vi "SerialTest.vi"(8 "error in (no error)":errorcluster, 11 "ControlBoard VISA":refnum<visa-resource-name>="ControlBoard") -> (0 "error out":errorcluster, 2 "Result":string="m\r\n\r\n\r\n----------------------------------------------\r\nEPC CONTROL BOARD TEST MENU: \r\n----------------------------------------------\r\na - Report ADC Results in Counts\r\nb - Repeat Single ADC Result\r\nc - Report ADC Results in Volts\r\nd - Clear Fault bits\r\ne - Report the Fault bits\r\nf - Run EEPROM Test\r\ng - Run SRAM Test\r\nh - Run Expansion Tests\r\ni - Turn Debug LEDs on/off\r\nj - Get Digital Input Pin State\r\nk - Set Digital Output Pin State\r\nl - Set Relay Driver State\r\nn - Boot Enable Pin State\r\no - Run CAN Test\r\np - Read QEP Input Bits\r\nq - Toggle Inverter A Output on/off\r\nr - Toggle Inverter B Output on/off\r\ns - Toggle Half Bridge Output on/off\r\nt - Set PWM leg duty cycle\r\nu - Real Time Clock\r\nv - Watchdog Control\r\nw - Test Interrupt Lines\r\nx - Read HALLs\r\ny - Test FPGA Read/Write\r\nz - Report Software/FPGA Revs\r\nm - Display this menu\r\n0 - Report Internal RAM Zeroed\r\n1 - Report SRAM Zeroed\r\n2 - Report SRAM Initialized\r\n3 - Run Quick EEPROM Test\r\n4 - Report Temperature and Humidity\r\n> ", 3 "Pass/Fail":bool)   [LabVIEW 2022 SP3]
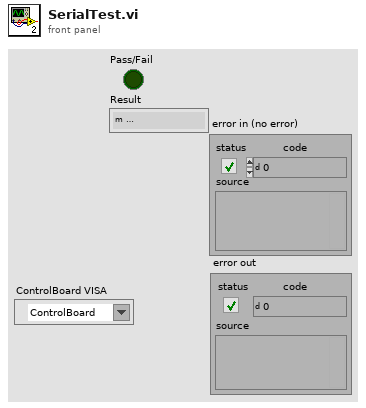
[diagram p1: front panel]
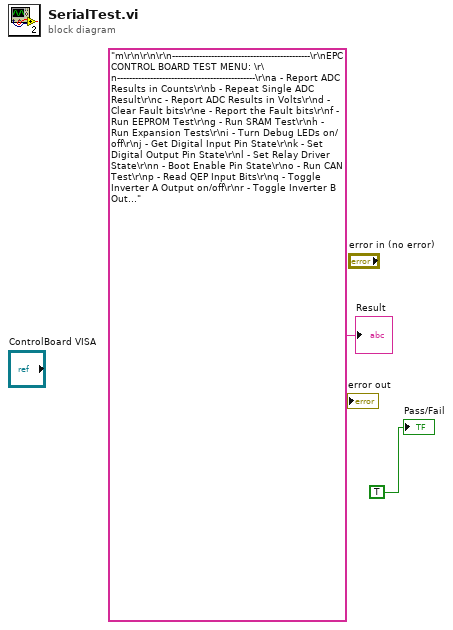
[diagram p0: block diagram]
diagram:
  "Pass/Fail" <- TRUE ("Pass/Fail 2")
  "Result" <- "m\r\n\r\n\r\n----------------------------------------------\r\nEPC CONTROL BOARD TEST MENU: \r\n----------------------------------------------\r\na - Report ADC Results in Counts\r\nb - Repeat Single ADC Result\r\nc - Report ADC Results in Volts\r\nd - Clear Fault bits\r\ne - Report the Fault bits\r\nf - Run EEPROM Test\r\ng - Run SRAM Test\r\nh - Run Expansion Tests\r\ni - Turn Debug LEDs on/off\r\nj - Get Digital Input Pin State\r\nk - Set Digital Output Pin State\r\nl - Set Relay Driver State\r\nn - Boot Enable Pin State\r\no - Run CAN Test\r\np - Read QEP Input Bits\r\nq - Toggle Inverter A Output on/off\r\nr - Toggle Inverter B Output on/off\r\ns - Toggle Half Bridge Output on/off\r\nt - Set PWM leg duty cycle\r\nu - Real Time Clock\r\nv - Watchdog Control\r\nw - Test Interrupt Lines\r\nx - Read HALLs\r\ny - Test FPGA Read/Write\r\nz - Report Software/FPGA Revs\r\nm - Display this menu\r\n0 - Report Internal RAM Zeroed\r\n1 - Report SRAM Zeroed\r\n2 - Report SRAM Initialized\r\n3 - Run Quick EEPROM Test\r\n4 - Report Temperature and Humidity\r\n> "
